vi "General Reading+Writing.vi"(8 "Write String":string, 9 "Bytes to Read":u32=2, 10 "VISA resource name":refnum<visa-resource-name>="COM6", 11 "String Seached":string) -> (0 "Coincidence Of Character":bool, 1 "Imag Data":i32[](array[numeric]), 2 "read buffer":string, 3 "Real Data":i32[](array[numeric]))   [LabVIEW 2011]
panel:
  out "error out":errorcluster
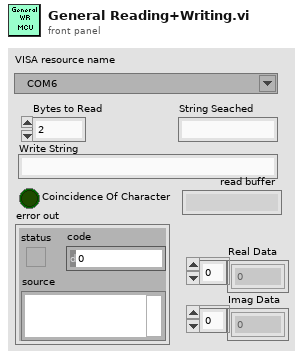
[diagram p1: front panel]
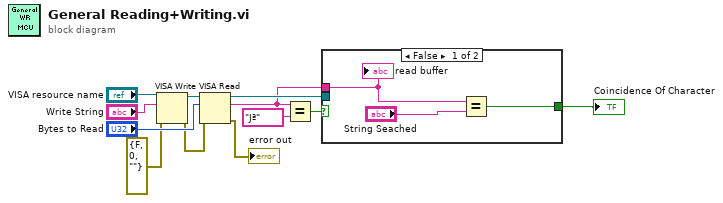
[diagram p0: block diagram]
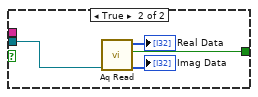
[diagram p2: hidden frame]
diagram:
  n1 = VISA Write(VISA resource name="VISA resource name", write buffer="Write String", error in (no error)=errorcluster {"status"=FALSE, "code"=0, "source"=""}) -> (VISA resource name out=w11:refnum<visa-resource-name>, error out=w2:errorcluster)  [unwired: 1 out]
  n2 = VISA Read(VISA resource name=w11, byte count="Bytes to Read", error in (no error)=w2) -> (VISA resource name out=w7:refnum<visa-resource-name>, read buffer=w6:string, error out=→"error out":errorcluster)  [unwired: 1 out]
  n3 = Equal?(x=w6, y="Jª" ("search string/char (-)")) -> (x = y?=w8:bool)
  n4 = case shown="False" w8 {
    tunnel: w7 -> [_ w19]
    tunnel: w6 -> [w15 _]
    tunnel: [w13 w18] -> w5
    frame False {
      n5 = Equal?(x=w15, y="String Seached") -> (x = y?=w13:bool)
      "read buffer" <- w15
    }
    frame True {
      n6 = call "Aq Read.vi"("VISA resource name"=w19) -> ("Imag Data"=→"Imag Data":i32[], "Coincidence Of Character"=w18:bool, "Real Data"=→"Real Data":i32[])  [unwired: 7 in, 1 out]
    }
  }
  "Coincidence Of Character" <- w5
